vi "Main_Control_working.vi"() -> ()   [LabVIEW 2016]
panel:
  out "Workspace":T1(tab)
  in  "s_Path":path caption="Path"
  out "Scan":picture
  out "s_InkScape_path":string caption="String"
  in  "b_Change_litho":bool caption="Change"
  in  "l_Litho_modes":i32(ring) caption="Tip Signal Mode" items=["Current Measurement ", "Voltage Source", "Direct from BNC"]
  in  "b_Lithography_Mode":bool caption="Blank"
  in  "b_Open_InkScape":bool caption="Open"
  in  "b_Save_Scan":bool caption="Save"
  in  "b_Config":bool caption="Config"
  # "InkScape should open momentarily.\nHowever, if it fails to load in a reasonable amount of time, below is the path of the InkScape file if needed"
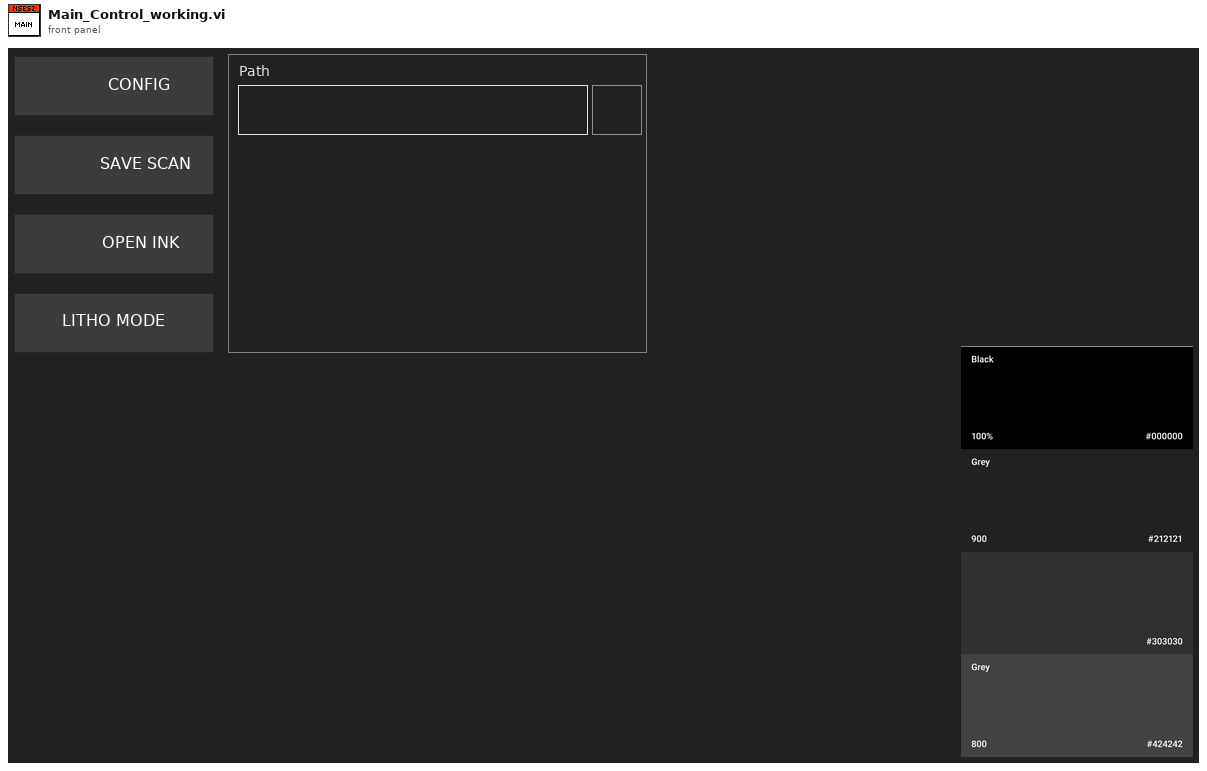
[diagram p1: front panel]
types:
  T1 = enum32{"CONFIG", "SAVE SCAN", "OPEN INKSCAPE", "LITHOMODE"}
  T2 = enum32{"invalid app kind", "Development System", "Run Time System", "Student Edition", "Embedded LabVIEW", "Evaluation", "Custom"}
  T3 = enum32{"Invalid", "Standard", "Closed", "Hidden", "Minimized", "Maximized"}
  T4 = cluster{"Core":cluster{"Current VI Reference":refnum<vi>, "Close Panel on Exit?":bool}, "Your Boolean data":bool, "Your string data":string, "Main_Path":path, "Image_Paths":cluster{"BMP":string, "BMP_Inkscape":string, "SVG_Inkscape":string}, "Application":refnum<k7>}
  T5 = cluster{"BMP":string, "BMP_Inkscape":string, "SVG_Inkscape":string}
  T6 = cluster{"Current VI Reference":refnum<vi>, "Close Panel on Exit?":bool}
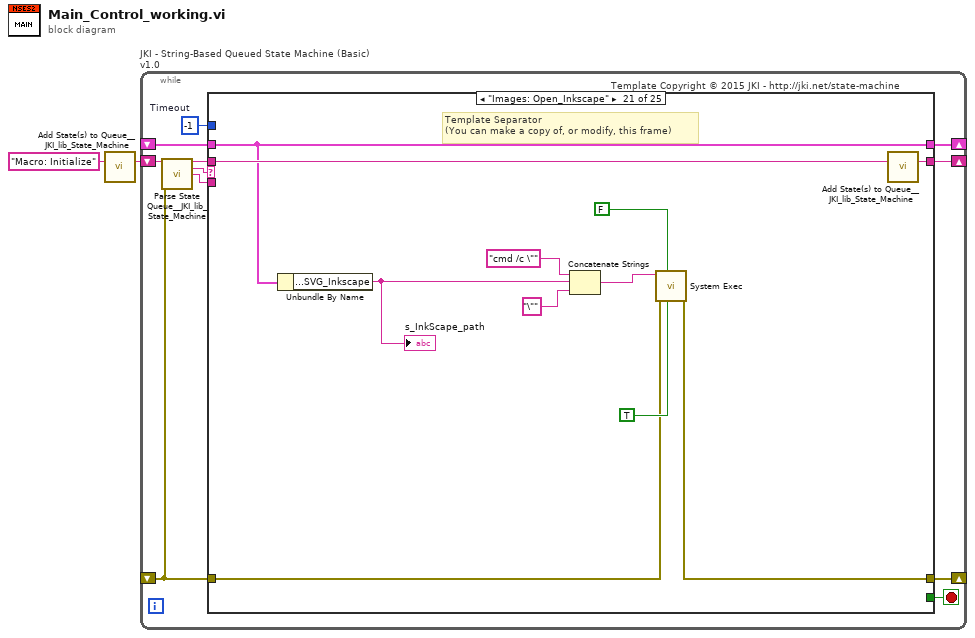
[diagram p0: block diagram]
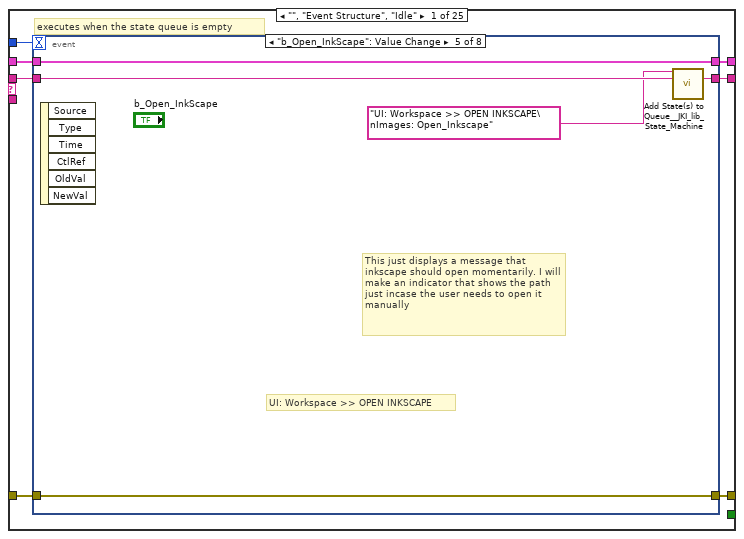
[diagram p2: hidden frame]
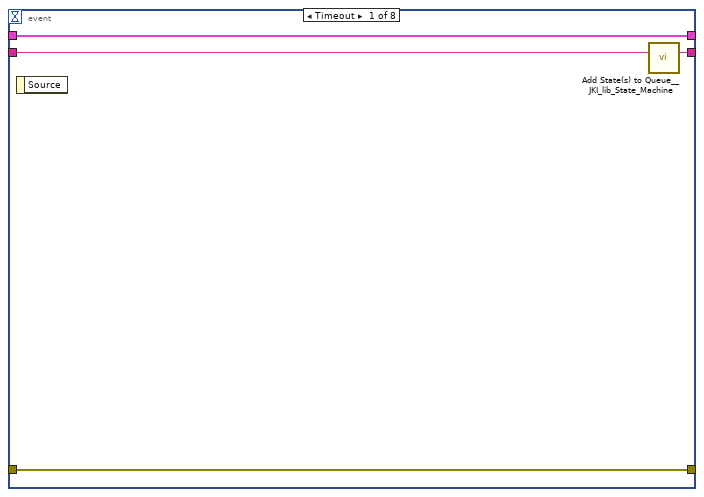
[diagram p3: hidden frame]
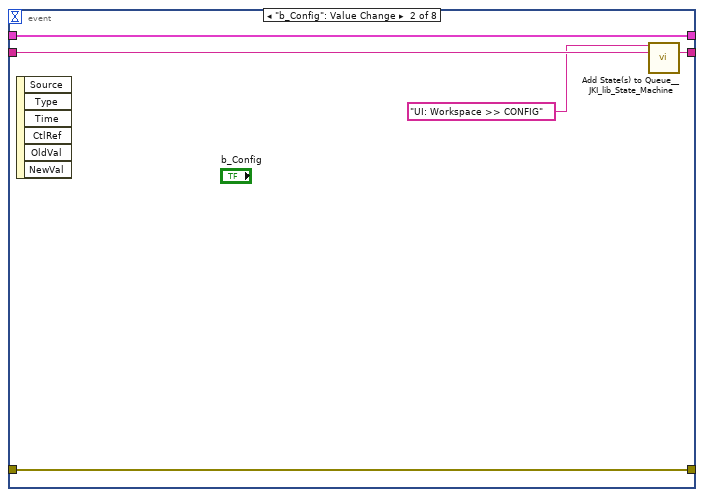
[diagram p4: hidden frame]
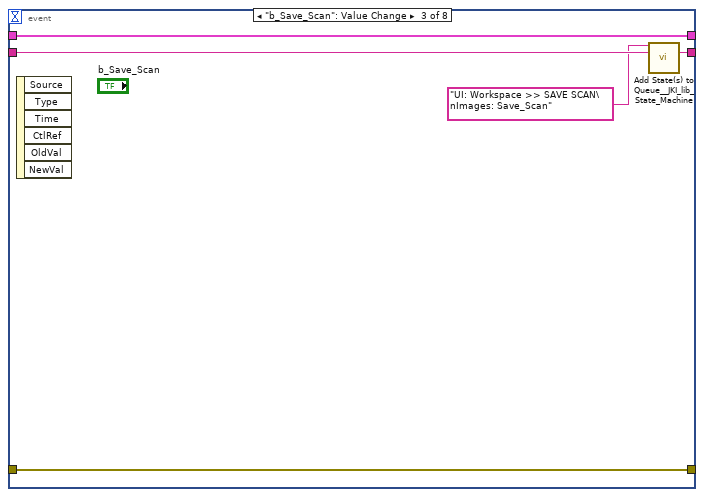
[diagram p5: hidden frame]
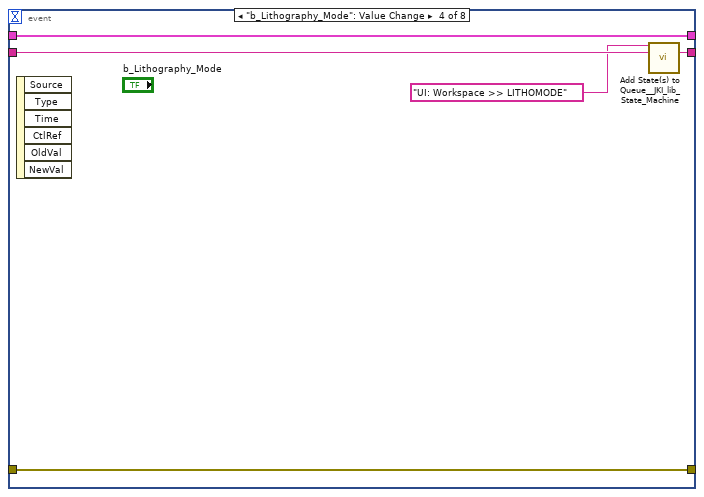
[diagram p6: hidden frame]
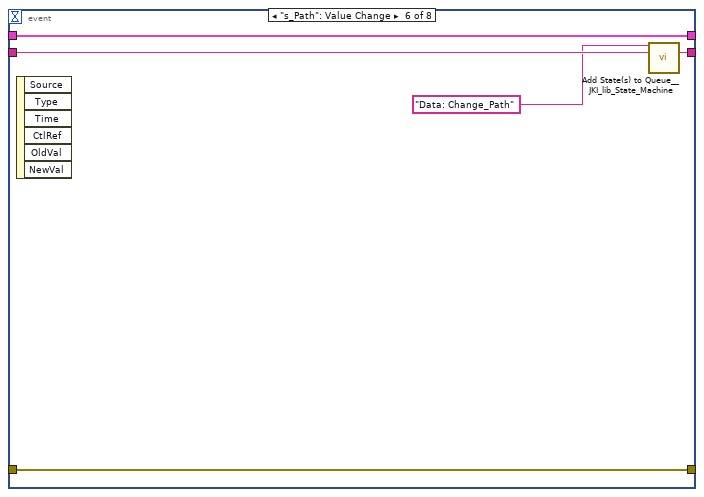
[diagram p7: hidden frame]
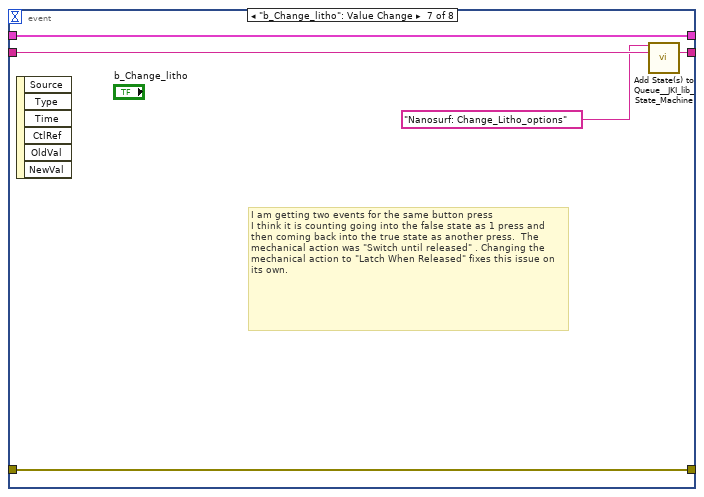
[diagram p8: hidden frame]
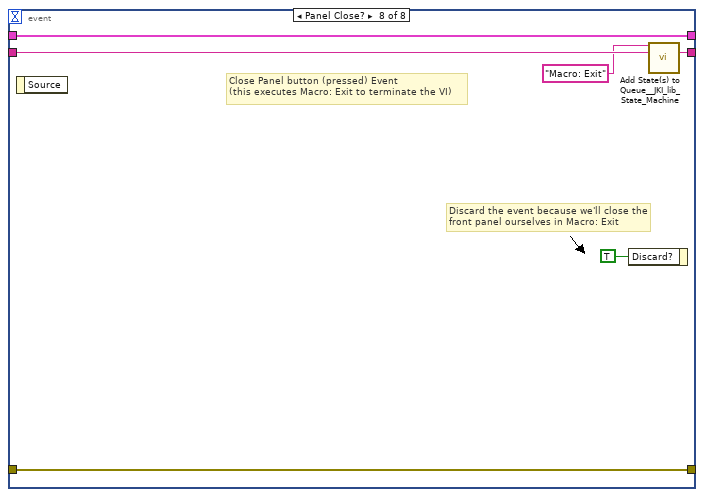
[diagram p9: hidden frame]
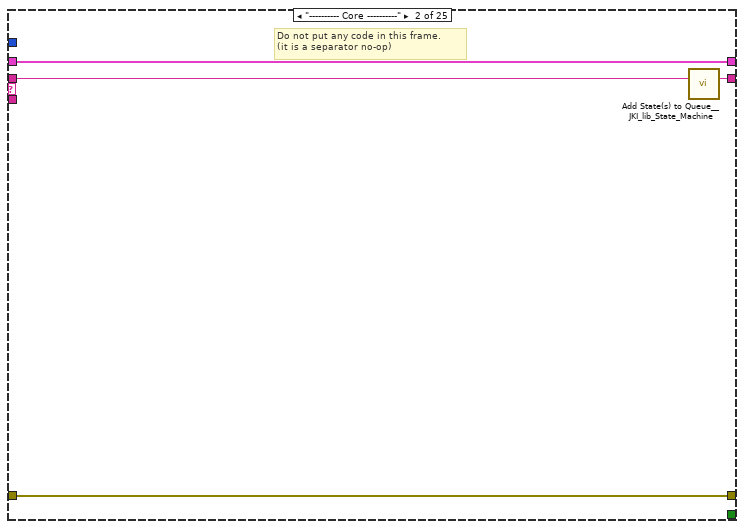
[diagram p10: hidden frame]
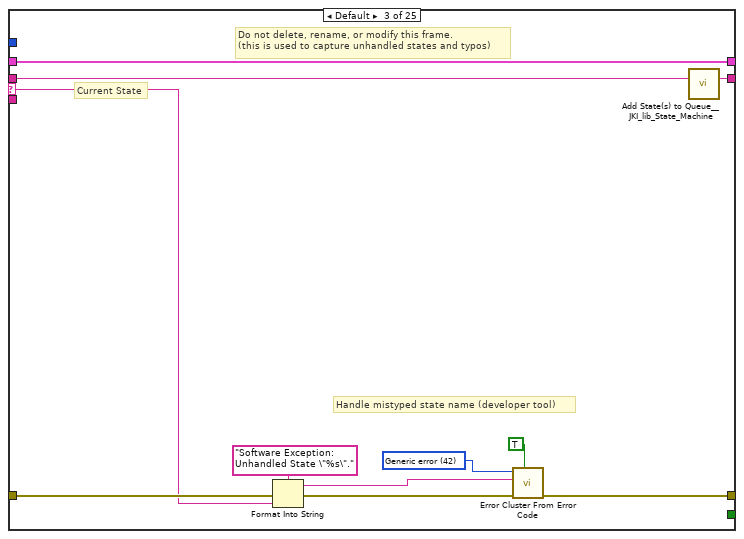
[diagram p11: hidden frame]
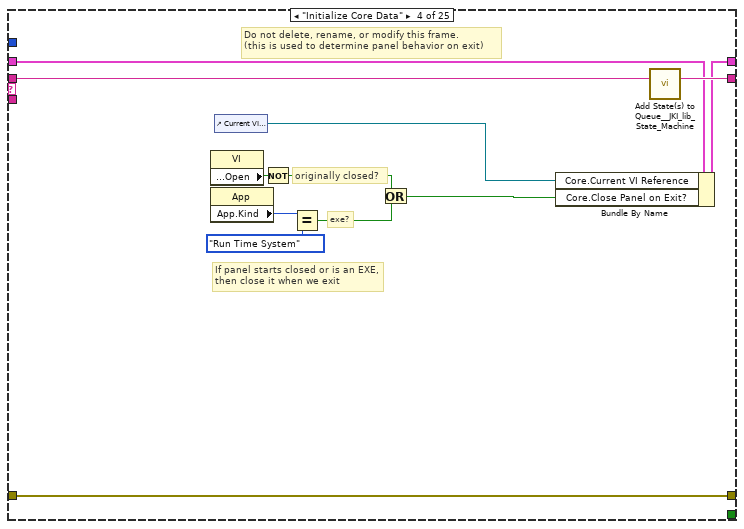
[diagram p12: hidden frame]
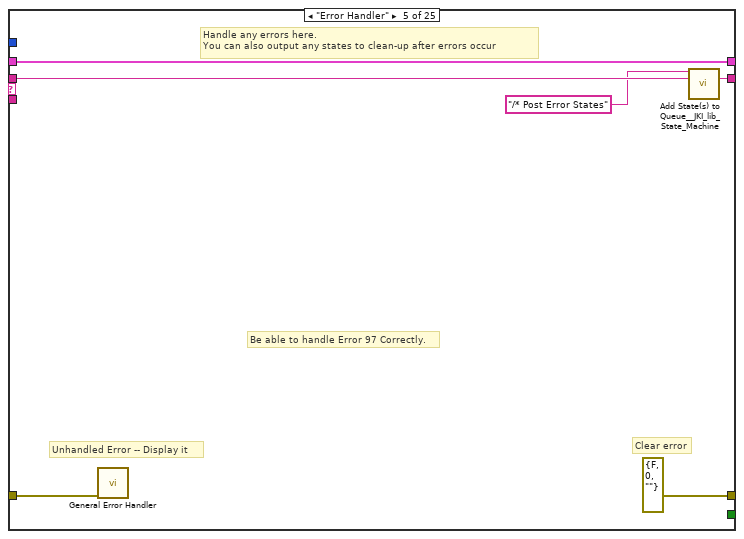
[diagram p13: hidden frame]
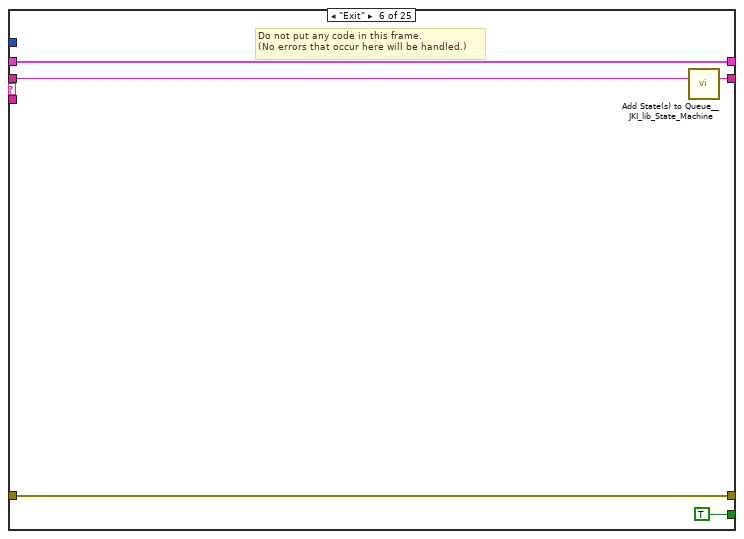
[diagram p14: hidden frame]
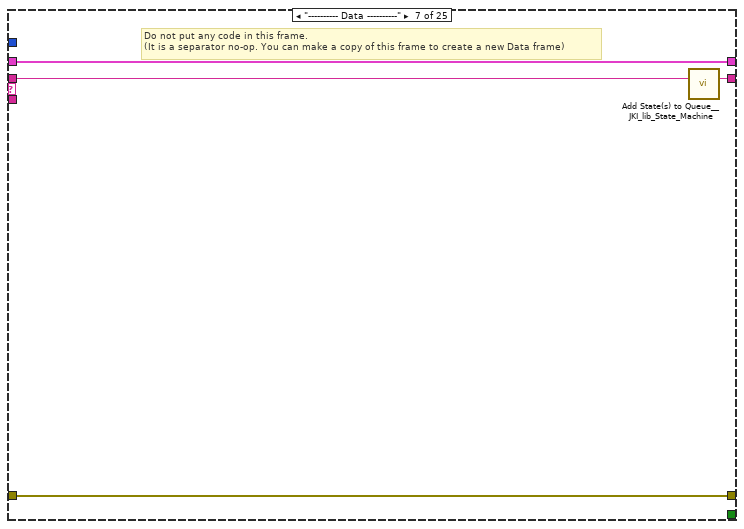
[diagram p15: hidden frame]
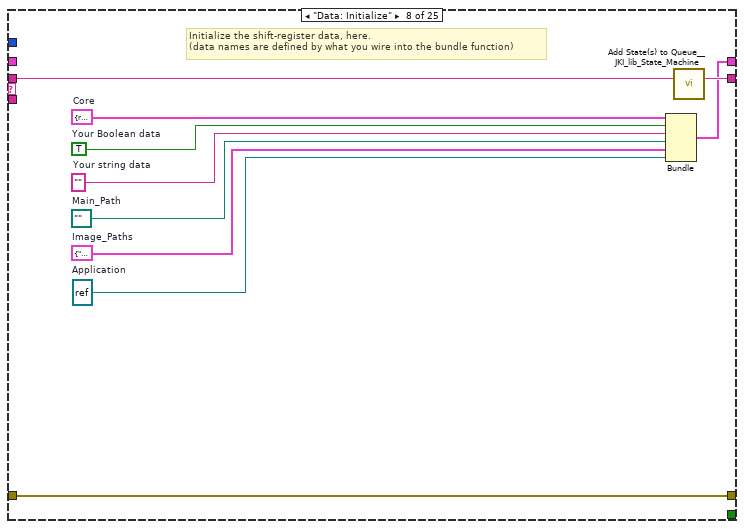
[diagram p16: hidden frame]
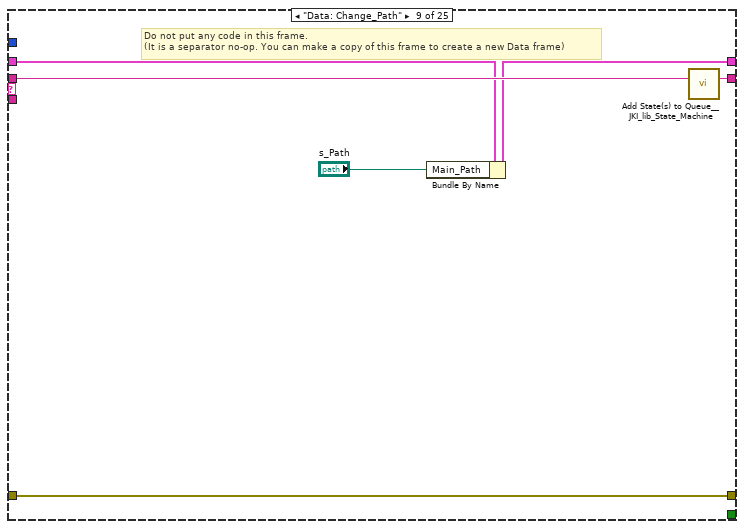
[diagram p17: hidden frame]
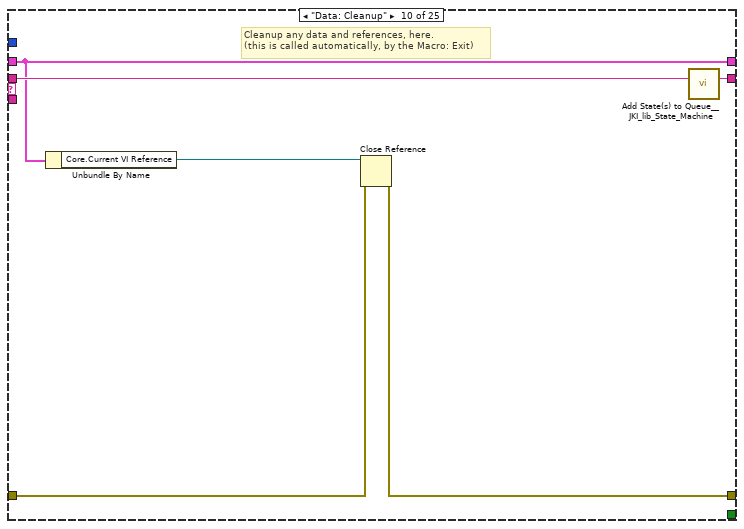
[diagram p18: hidden frame]
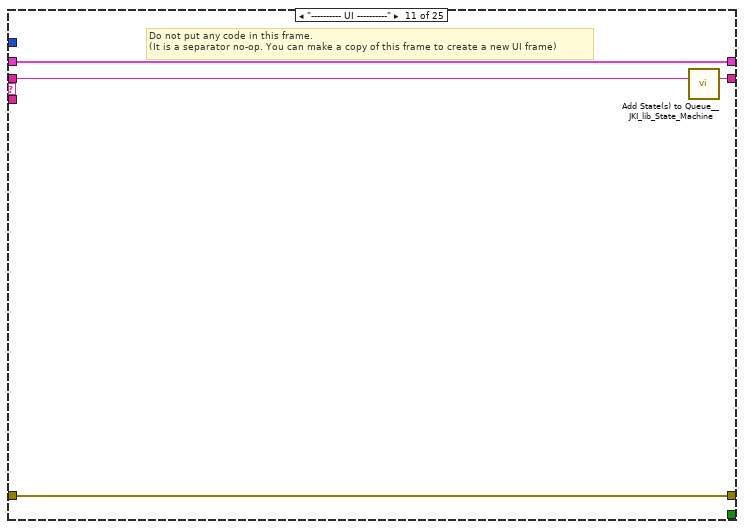
[diagram p19: hidden frame]
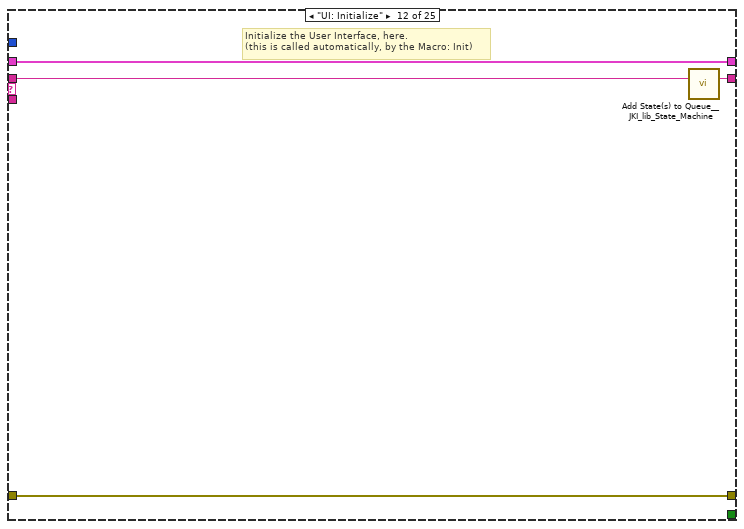
[diagram p20: hidden frame]
diagram:
  n1 = call <vilib>:"Add State(s) to Queue__JKI_lib_State_Machine.vi"("State(s) in (\"\")"="Macro: Initialize") -> ("States Out"=w2:string)  [unwired: 14 in]
  n2 = while "JKI - String-Based Queued State Machine (Basic) v1.0" {
    shift-right: [w6] -> _
    shift-left: _ -> [w5]
    shift-right: [w9] -> _
    shift-left: _ -> [w3]
    shift-right: [w8] -> _
    shift-left: w2 -> [w10]
    stop <- w7 stop-if-true
    w4 = -1  # Timeout
    # "Template Copyright © 2015 JKI - http://jki.net/state-machine"
    n3 = call <vilib>:"Parse State Queue__JKI_lib_State_Machine.vi"("State Queue"=w10, "Error In (no error)"=w3) -> ("Remaining States"=w12:string, "Current State"=w13:string, "Arguments"=w11:string)  [unwired: 11 in]
    n4 = case shown="\"Images: Open_Inkscape\"" w13 {
      selector: w13 -> [_ _ w65 _ _ _ _ _ _ _ _ _ _ _ _ _ _ _ _ _ _ _ _ _ _]
      tunnel: w12 -> [w20 w64 w69 w87 w93 w98 w102 w112 w118 w124 w128 w132 w138 w149 w177 w185 w190 w200 w204 w217 w228 w232 w240 w247 w253]
      tunnel: w11 -> [_ _ _ _ _ _ _ _ _ _ _ _ w133 w143 w173 _ _ _ _ _ _ _ _ _ _]
      tunnel: w5 -> [w18 w61 w67 w78 w90 w96 w99 _ w115 w119 w125 w130 w136 w145 w174 w182 w187 w197 w202 w210 w219 w229 w234 w245 w249]
      tunnel: [w17 w62 w71 w84 errorcluster {"status"=FALSE, "code"=0, "source"=""} ("error out") w95 w100 w109 w116 w120 w126 w129 w134 w146 w175 w183 w188 w198 w201 w213 w220 w230 w236 w241 w250] -> w9
      tunnel: w3 -> [w16 w62 w70 w84 w89 w95 w100 w109 w116 w121 w126 w129 w135 w147 w175 w183 w188 w198 w201 w214 w221 w230 w237 w242 w251]
      tunnel: [w19 w63 w68 w86 w92 w97 w101 w111 w117 w123 w127 w131 w137 w148 w176 w184 w189 w199 w203 w216 w227 w231 w239 w246 w252] -> w8
      tunnel: [_ _ _ _ _ TRUE _ _ _ _ _ _ _ _ _ _ _ _ _ _ _ _ _ _ _] -> w7
      tunnel: [w15 w61 w67 w85 w90 w96 w99 w110 w114 w119 w125 w130 w136 w145 w174 w182 w187 w197 w202 w209 w219 w229 w233 w245 w249] -> w6
      tunnel: w4 -> [w14 _ _ _ _ _ _ _ _ _ _ _ _ _ _ _ _ _ _ _ _ _ _ _ _]
      frame "", "Event Structure", "Idle" {
        # "executes when the state queue is empty"
        n5 = event shown="[4] \"b_Open_InkScape\": Value Change" {
          selector: _ -> [_ _ _ _ _ _ _ _]
          dyn-events: _ -> [_ _ _ _ _ _ _ _]
          timeout: w14 -> [_ _ _ _ _ _ _ _]
          tunnel: w20 -> [w24 w29 w34 w39 w44 w49 w54 w60]
          tunnel: [w23 w28 w33 w38 w43 w48 w53 w59] -> w19
          tunnel: w18 -> [w21 w26 w31 w36 w41 w46 w51 w57]
          tunnel: [w22 w27 w32 w37 w42 w47 w52 w58] -> w17
          tunnel: w16 -> [w22 w27 w32 w37 w42 w47 w52 w58]
          tunnel: [w21 w26 w31 w36 w41 w46 w51 w57] -> w15
          event Timeout {
            n6 = event-data() -> ()  [unwired: 1 in, 1 out]
            n7 = call <vilib>:"Add State(s) to Queue__JKI_lib_State_Machine.vi"("State(s) in (\"\")"=w24) -> ("States Out"=w23:string)  [unwired: 14 in]
          }
          event "b_Config": Value Change {
            n8 = event-data() -> ()  [unwired: 1 in, 6 out]
            n9 = call <vilib>:"Add State(s) to Queue__JKI_lib_State_Machine.vi"("State(s) in Front (\"\")"="UI: Workspace >> CONFIG" ("State(s) in Front (\"\")"), "State(s) in (\"\")"=w29) -> ("States Out"=w28:string)  [unwired: 13 in]
          }
          event "b_Save_Scan": Value Change {
            n10 = event-data() -> ()  [unwired: 1 in, 6 out]
            n11 = call <vilib>:"Add State(s) to Queue__JKI_lib_State_Machine.vi"("State(s) in Front (\"\")"="UI: Workspace >> SAVE SCAN\nImages: Save_Scan" ("State(s) in Front (\"\")"), "State(s) in (\"\")"=w34) -> ("States Out"=w33:string)  [unwired: 13 in]
          }
          event "b_Lithography_Mode": Value Change {
            n12 = event-data() -> ()  [unwired: 1 in, 6 out]
            n13 = call <vilib>:"Add State(s) to Queue__JKI_lib_State_Machine.vi"("State(s) in Front (\"\")"="UI: Workspace >> LITHOMODE" ("State(s) in Front (\"\")"), "State(s) in (\"\")"=w39) -> ("States Out"=w38:string)  [unwired: 13 in]
          }
          event "b_Open_InkScape": Value Change {
            # "This just displays a message that inkscape should open momentarily. I will make an indicator that shows the path just incase the user needs to open it manually"
            # "UI: Workspace >> OPEN INKSCAPE"
            n14 = event-data() -> ()  [unwired: 1 in, 6 out]
            n15 = call <vilib>:"Add State(s) to Queue__JKI_lib_State_Machine.vi"("State(s) in Front (\"\")"="UI: Workspace >> OPEN INKSCAPE\nImages: Open_Inkscape" ("State(s) in Front (\"\")"), "State(s) in (\"\")"=w44) -> ("States Out"=w43:string)  [unwired: 13 in]
          }
          event "s_Path": Value Change {
            n16 = event-data() -> ()  [unwired: 1 in, 6 out]
            n17 = call <vilib>:"Add State(s) to Queue__JKI_lib_State_Machine.vi"("State(s) in Front (\"\")"="Data: Change_Path" ("State(s) in Front (\"\")"), "State(s) in (\"\")"=w49) -> ("States Out"=w48:string)  [unwired: 13 in]
          }
          event "b_Change_litho": Value Change {
            # "I am getting two events for the same button press \nI think it is counting going into the false state as 1 press and then coming back into the true state as another press.  The mechanical action was \"Switch until released\" . Changing the mechanical action to \"Latch When Released\" fixes this issue on its own."
            n18 = event-data() -> ()  [unwired: 1 in, 6 out]
            n19 = call <vilib>:"Add State(s) to Queue__JKI_lib_State_Machine.vi"("State(s) in Front (\"\")"="Nanosurf: Change_Litho_options", "State(s) in (\"\")"=w54) -> ("States Out"=w53:string)  [unwired: 13 in]
          }
          event Panel Close? {
            # "Discard the event because we'll close the front panel ourselves in Macro: Exit"
            # "Close Panel button (pressed) Event\n(this executes Macro: Exit to terminate the VI)"
            n20 = event-data() -> ()  [unwired: 1 in, 1 out]
            n21 = event-data("Discard?"=TRUE) -> ()  [unwired: 1 in, 1 out]
            n22 = call <vilib>:"Add State(s) to Queue__JKI_lib_State_Machine.vi"("State(s) in Front (\"\")"="Macro: Exit", "State(s) in (\"\")"=w60) -> ("States Out"=w59:string)  [unwired: 13 in]
          }
        }
      }
      frame "---------- Core ----------" {
        # "Do not put any code in this frame.\n(it is a separator no-op)"
        n23 = call <vilib>:"Add State(s) to Queue__JKI_lib_State_Machine.vi"("State(s) in (\"\")"=w64) -> ("States Out"=w63:string)  [unwired: 14 in]
      }
      frame Default {
        w74 = 42 items=["No error", "Argument error", "Memory is full", "Out of zone", "End of file", "File already open", "Generic file I/O error", "File not found", "File permission error", "Disk is full", "Duplicate path", "Too many files open", "System feature not enabled", "Resource file not found", "Cannot add resource", "Resource not found", "Image not found", "Image memory error", "Pen does not exist", "Config type invalid", "Config token not found", "Config parse error", "Config memory error", "Bad external code format", "Bad external code offset", "External code not present", "Null window", "Destroy window error", "Null menu", "Print aborted", "Bad print record", "Print driver error", "Windows error during printing", "Memory error during printing", "Print dialog error", "Generic print error", "Invalid device refnum", "Device not found", "Device parameter error", "Device unit error", "Cannot open device", "Device call aborted", "Generic error", "Cancelled by user", "Object ID too low", "Object ID too high", "Object not in heap", "Unknown heap", "Unknown object (invalid DefProc)", "Unknown object (DefProc not in table)", "Message out of range", "Invalid (null) method", "Unknown message", "Manager call not supported", "Bad address", "Network operation in progress", "Network operation timed out", "Connection is busy", "Network attribute not supported", "Network error", "Address in use", "System out of memory", "Connection aborted", "Connection refused", "Not connected", "Already connected", "Connection closed", "Initialization error (interapplication manager)", "Bad occurrence", "Wait on unbound occurrence handler", "Occurrence queue overflow", "Datalog type conflict", "Unused", "Unrecognized type (interapplication manager)", "Memory corrupt", "Failed to make temporary DLL", "Old CIN version", "Drag socket not found", "Failed to load drop-object", "Failed to register OLE object", "Failed to release OLE object", "Format specifier type mismatch", "Unknown format specifier", "Too few format specifiers", "Too many format specifiers", "Scan failed", "Newer CIN version", "Error converting to variant", "Runtime menu error", "Password tampered", "Variant attribute not found", "Incompatible variant data type", "Event data is not available", "Event Store is not present", "Occurrence is not found", "Event Queue is not created", "Event info is not available", "Refnum passed is NULL", "Error retrieving Class GUID", "Error retrieving CoClass GUID", "Error retrieving TypeLib GUID.", "Bad built application magic bytes.", "Specific driver is different from the specific driver associated with the Logical Name.", "There is no session opened to the class driver.", "Max Error", "MAX - Error with config objects", "MAX - Error loading configuration", "MAX - Group not supported"]
        # "Current State"
        # "Do not delete, rename, or modify this frame.\n(this is used to capture unhandled states and typos)"
        # "Handle mistyped state name (developer tool)"
        n24 = Format Into String(format string="Software Exception: Unhandled State \"%s\"." ("message"), error in=w70, w65) -> (resulting string=w73:string, error out=w72:errorcluster)  [unwired: 1 in]
        n25 = call <vilib>:"Error Cluster From Error Code.vi"("show call chain? (False)"=TRUE, "error in (no error)"=w72, "error message (\"\")"=w73, "error code (0)"=w74) -> ("error out"=w71:errorcluster)  [unwired: 5 in]
        n26 = call <vilib>:"Add State(s) to Queue__JKI_lib_State_Machine.vi"("State(s) in (\"\")"=w69) -> ("States Out"=w68:string)  [unwired: 14 in]
      }
      frame "Initialize Core Data" {
        # "Do not delete, rename, or modify this frame.\n(this is used to determine panel behavior on exit)"
        # "originally closed?"
        # "exe?"
        # "If panel starts closed or is an EXE, then close it when we exit"
        n27 = property class="VI"() -> ("Front Panel.Open"=w83:bool)  [unwired: 2 in, 2 out]
        n28 = property class="App"() -> ("App.Kind"=w82:T2)  [unwired: 2 in, 2 out]
        n29 = control-ref of="Current VI Reference"() -> (w76:refnum<vi>)
        n30 = Not(x=w83) -> (.not. x?=w80:bool)
        n31 = Equal?(x=w82, y=T2."Run Time System" ("Application:Kind")) -> (x = y?=w79:bool)
        n32 = Or(x=w80, y=w79) -> (x .or. y?=w77:bool)
        n33 = Bundle By Name(cluster=w78, "Core.Current VI Reference"=w76, "Core.Close Panel on Exit?"=w77) -> (w85:T4)
        n34 = call <vilib>:"Add State(s) to Queue__JKI_lib_State_Machine.vi"("State(s) in (\"\")"=w87) -> ("States Out"=w86:string)  [unwired: 14 in]
      }
      frame "Error Handler" {
        # "Be able to handle Error 97 Correctly."
        # "Unhandled Error -- Display it"
        # "Handle any errors here.\nYou can also output any states to clean-up after errors occur"
        # "Clear error"
        n35 = call <vilib>:"General Error Handler.vi"("error in (no error)"=w89) -> ()  [unwired: 10 in, 5 out]
        n36 = call <vilib>:"Add State(s) to Queue__JKI_lib_State_Machine.vi"("State(s) in Front (\"\")"="/* Post Error States", "State(s) in (\"\")"=w93) -> ("States Out"=w92:string)  [unwired: 13 in]
      }
      frame "Exit" {
        # "Do not put any code in this frame.\n(No errors that occur here will be handled.)"
        n37 = call <vilib>:"Add State(s) to Queue__JKI_lib_State_Machine.vi"("State(s) in (\"\")"=w98) -> ("States Out"=w97:string)  [unwired: 14 in]
      }
      frame "---------- Data ----------" {
        # "Do not put any code in this frame.\n(It is a separator no-op. You can make a copy of this frame to create a new Data frame)"
        n38 = call <vilib>:"Add State(s) to Queue__JKI_lib_State_Machine.vi"("State(s) in (\"\")"=w102) -> ("States Out"=w101:string)  [unwired: 14 in]
      }
      frame "Data: Initialize" {
        w103 = refnum<k7> refnum  # Application
        w104 = T5 {"BMP"="", "BMP_Inkscape"="", "SVG_Inkscape"=""}  # Image_Paths
        w105 = path ""  # Main_Path
        w106 = T6 {"Current VI Reference"=refnum, "Close Panel on Exit?"=FALSE}  # Core
        w108 = TRUE  # Your Boolean data
        w107 = ""  # Your string data
        # "Initialize the shift-register data, here.\n(data names are defined by what you wire into the bundle function)"
        n39 = Bundle("Core"=w106, "Your Boolean data"=w108, "Your string data"=w107, "Main_Path"=w105, "Image_Paths"=w104, "Application"=w103) -> (w110:T4)  [unwired: 1 in]
        n40 = call <vilib>:"Add State(s) to Queue__JKI_lib_State_Machine.vi"("State(s) in (\"\")"=w112) -> ("States Out"=w111:string)  [unwired: 14 in]
      }
      frame "Data: Change_Path" {
        # "Do not put any code in this frame.\n(It is a separator no-op. You can make a copy of this frame to create a new Data frame)"
        n41 = Bundle By Name(cluster=w115, "Main_Path"="s_Path") -> (w114:T4)
        n42 = call <vilib>:"Add State(s) to Queue__JKI_lib_State_Machine.vi"("State(s) in (\"\")"=w118) -> ("States Out"=w117:string)  [unwired: 14 in]
      }
      frame "Data: Cleanup" {
        # "Cleanup any data and references, here.\n(this is called automatically, by the Macro: Exit)"
        n43 = Unbundle By Name(w119) -> ("Core.Current VI Reference"=w122:refnum<vi>)
        n44 = Close Reference(reference=w122, error in (no error)=w121) -> (error out=w120:errorcluster)
        n45 = call <vilib>:"Add State(s) to Queue__JKI_lib_State_Machine.vi"("State(s) in (\"\")"=w124) -> ("States Out"=w123:string)  [unwired: 14 in]
      }
      frame "---------- UI ----------" {
        # "Do not put any code in this frame.\n(It is a separator no-op. You can make a copy of this frame to create a new UI frame)"
        n46 = call <vilib>:"Add State(s) to Queue__JKI_lib_State_Machine.vi"("State(s) in (\"\")"=w128) -> ("States Out"=w127:string)  [unwired: 14 in]
      }
      frame "UI: Initialize" {
        # "Initialize the User Interface, here.\n(this is called automatically, by the Macro: Init)"
        n47 = call <vilib>:"Add State(s) to Queue__JKI_lib_State_Machine.vi"("State(s) in (\"\")"=w132) -> ("States Out"=w131:string)  [unwired: 14 in]
      }
      frame "UI: Cursor Set" {
        # "Argument"
        # "Set and Unset Cursor Busy.\n(Usage: \"UI: Cursor Set >> Busy|Idle\")"
        n48 = case shown="\"Idle\", Default" w133 {
          tunnel: w135 -> [w140 w142]
          tunnel: [w139 w141] -> w134
          frame "Idle", Default {
            n49 = call <vilib>:"Unset Busy.vi"("error in (no error)"=w140) -> ("error out"=w139:errorcluster)  [unwired: 10 in]
          }
          frame "Busy" {
            n50 = call <vilib>:"Set Busy.vi"("error in (no error)"=w142) -> ("error out"=w141:errorcluster)  [unwired: 9 in, 1 out]
          }
        }
        n51 = call <vilib>:"Add State(s) to Queue__JKI_lib_State_Machine.vi"("State(s) in (\"\")"=w138) -> ("States Out"=w137:string)  [unwired: 14 in]
      }
      frame "UI: Front Panel State" {
        # "Argument"
        # "Set Front Panel Open or Closed\n(Usage: \"UI: Front Panel State >> Open|Close\")"
        n52 = Unbundle By Name(w145) -> ("Core.Current VI Reference"=w144:refnum<vi>)
        n53 = case shown="\"Open\", Default" w143 {
          tunnel: w147 -> [w153 w166]
          tunnel: [w155 w167] -> w146
          tunnel: w144 -> [w154 w164]
          frame "Open", Default {
            n54 = property class="VI"(reference=w154, error in=w153) -> (reference out=w151:refnum<vi>, error out=w152:errorcluster, "Front Panel.Open"=w150:bool)
            n55 = case shown="False" w150 {
              tunnel: [w158 w161] -> w155
              tunnel: w152 -> [w157 w161]
              tunnel: w151 -> [w156 _]
              frame False {
                n56 = invoke class="VI" method="FP.Open"(reference=w156, error in=w157, "Activate"=TRUE, "State"=T3."Standard") -> (error out=w158:errorcluster)  [unwired: 1 in, 4 out]
              }
              frame True {
              }
            }
          }
          frame "Close" {
            n57 = property class="VI"(reference=w164, error in=w166) -> (reference out=w163:refnum<vi>, error out=w165:errorcluster, "Front Panel.Open"=w162:bool)
            n58 = case shown="True" w162 {
              tunnel: [w168 w171] -> w167
              tunnel: w165 -> [w168 w170]
              tunnel: w163 -> [_ w169]
              frame False {
              }
              frame True {
                n59 = invoke class="VI" method="FP.Close"(reference=w169, error in=w170) -> (error out=w171:errorcluster)  [unwired: 1 in, 2 out]
              }
            }
          }
        }
        n60 = call <vilib>:"Add State(s) to Queue__JKI_lib_State_Machine.vi"("State(s) in (\"\")"=w149) -> ("States Out"=w148:string)  [unwired: 14 in]
      }
      frame "UI: Workspace" {
        # "Workspace Tab State\n(This is the frame that changes the Workspace Value)"
        n61 = case shown="\"OPEN INKSCAPE\"" w173 {
          tunnel: [T1."CONFIG" ("Workspace") T1."SAVE SCAN" ("Workspace") T1."OPEN INKSCAPE" ("Workspace") T1."LITHOMODE" ("Workspace")] -> w172
          frame "CONFIG", Default {
            # "UI: Workspace >> CONFIG"
          }
          frame "SAVE SCAN" {
            # "UI: Workspace >> SAVE SCAN"
          }
          frame "OPEN INKSCAPE" {
            # "UI: Workspace >> OPEN INKSCAPE"
          }
          frame "LITHOMODE" {
            # "UI: Workspace >> LITHOMODE"
          }
        }
        "Workspace" <- w172
        n62 = call <vilib>:"Add State(s) to Queue__JKI_lib_State_Machine.vi"("State(s) in (\"\")"=w177) -> ("States Out"=w176:string)  [unwired: 14 in]
      }
      frame "---------- Macro ----------" {
        # "Do not put any code in this frame.\n(It is a separator no-op. You can make a copy of this frame to create a new Macro frame)"
        n63 = call <vilib>:"Add State(s) to Queue__JKI_lib_State_Machine.vi"("State(s) in (\"\")"=w185) -> ("States Out"=w184:string)  [unwired: 14 in]
      }
      frame "Macro: Initialize" {
        w186 = "Data: Initialize\nInitialize Core Data\nUI: Initialize\nUI: Front Panel State >> Open\nUI: Workspace >> CONFIG\nNanosurf: Open_Application\nData: Change_Path"  # Data: Initialize Initialize Core Data UI: Initialize UI: Front Panel State >> Open UI: Workspace >> CONFIG Nanosurf: Open_Application Data: Change_Path
        # "Initialization Macro\n(This is called once, when the VI starts)"
        n64 = call <vilib>:"Add State(s) to Queue__JKI_lib_State_Machine.vi"("State(s) in Front (\"\")"=w186, "State(s) in (\"\")"=w190) -> ("States Out"=w189:string)  [unwired: 13 in]
      }
      frame "Macro: Exit" {
        # "Exit Macro\n(This is called once, when the VI exits)"
        n65 = Unbundle By Name(w197) -> ("Core.Close Panel on Exit?"=w196:bool)
        n66 = Select(t="UI: Front Panel State >> Close", s=w196, f="") -> (s? t:f=w193:string)
        n67 = call <vilib>:"Add State(s) to Queue__JKI_lib_State_Machine.vi"("State(s) in (\"\")"=w193, "State(s) at Back (\"\")"="UI: Workspace >> CONFIG\nNanosurf: Close_Application\nData: Cleanup\nExit") -> ("States Out"=w191:string)  [unwired: 13 in]
        n68 = call <vilib>:"Add State(s) to Queue__JKI_lib_State_Machine.vi"("State(s) in Front (\"\")"=w191, "State(s) in (\"\")"=w200) -> ("States Out"=w199:string)  [unwired: 13 in]
      }
      frame "---------- Images ----------" {
        # "Template Separator\n(You can make a copy of, or modify, this frame)"
        n69 = call <vilib>:"Add State(s) to Queue__JKI_lib_State_Machine.vi"("State(s) in (\"\")"=w204) -> ("States Out"=w203:string)  [unwired: 14 in]
      }
      frame "Images: Save_Scan" {
        # "Template Separator\n(This will make an make a copy of, or modify, this frame)"
        n70 = Unbundle By Name(w210) -> ("Application"=w205:refnum<k7>, "Main_Path"=w211:path)
        n71 = call "Generic file paths.vi"("error in (no error)"=w214, "Parent Folder"=w211) -> ("error out"=w215:errorcluster, "SVG Path"=w206:string, "BMP for inkscape path"=w207:string, "BMP Path"=w208:string)  [unwired: 6 in]
        n72 = call "Save_Scan_macro.vi"("Application"=w205, "error in (no error)"=w215, "InkScape"=w206, "BMP INK Path"=w207, "BMP Path"=w208) -> ("error out"=w213:errorcluster, "BMP"=→"Scan":picture)  [unwired: 5 in]
        n73 = Bundle By Name(cluster=w210, "Image_Paths.BMP"=w208, "Image_Paths.BMP_Inkscape"=w207, "Image_Paths.SVG_Inkscape"=w206) -> (w209:T4)
        n74 = call <vilib>:"Add State(s) to Queue__JKI_lib_State_Machine.vi"("State(s) in (\"\")"=w217) -> ("States Out"=w216:string)  [unwired: 14 in]
      }
      frame "Images: Open_Inkscape" {
        # "Template Separator\n(You can make a copy of, or modify, this frame)"
        n75 = Unbundle By Name(w219) -> ("Image_Paths.SVG_Inkscape"=w218:string)
        "s_InkScape_path" <- w218
        n76 = Concatenate Strings("cmd /c \"", w218, "\"") -> (w224:string)
        n77 = call <vilib>:"System Exec.vi"("run minimized? (F)"=TRUE, "wait until completion? (T)"=FALSE, "error in (no error)"=w221, "command line"=w224) -> ("error out"=w220:errorcluster)  [unwired: 4 in, 3 out]
        n78 = call <vilib>:"Add State(s) to Queue__JKI_lib_State_Machine.vi"("State(s) in (\"\")"=w228) -> ("States Out"=w227:string)  [unwired: 14 in]
      }
      frame "---------- Nanosurf ----------" {
        # "Template Separator\n(You can make a copy of, or modify, this frame)"
        n79 = call <vilib>:"Add State(s) to Queue__JKI_lib_State_Machine.vi"("State(s) in (\"\")"=w232) -> ("States Out"=w231:string)  [unwired: 14 in]
      }
      frame "Nanosurf: Open_Application" {
        n80 = Unbundle By Name(w234) -> ("Application"=w238:refnum<k7>)
        n81 = Automation Open(error in (no error)=w237, Automation Refnum=w238) -> (Automation Refnum=w235:refnum<k7>, error out=w236:errorcluster)  [unwired: 2 in]
        n82 = Bundle By Name(cluster=w234, "Application"=w235) -> (w233:T4)
        n83 = call <vilib>:"Add State(s) to Queue__JKI_lib_State_Machine.vi"("State(s) in (\"\")"=w240) -> ("States Out"=w239:string)  [unwired: 14 in]
      }
      frame "Nanosurf: Change_Litho_options" {
        # "Change Lithography Options\n(Changes what the microscope uses to source the tip voltage. [more options may be added later])"
        n84 = Unbundle By Name(w245) -> ("Application"=w244:refnum<k7>)
        n85 = call "Change_tip_signal.vi"("error in (no error)"=w242, "l_Litho_modes"="l_Litho_modes", "Application"=w244) -> ("error out"=w241:errorcluster)  [unwired: 8 in]
        n86 = call <vilib>:"Add State(s) to Queue__JKI_lib_State_Machine.vi"("State(s) in (\"\")"=w247) -> ("States Out"=w246:string)  [unwired: 14 in]
      }
      frame "Nanosurf: Close_Application" {
        # "Template Separator\n(You can make a copy of, or modify, this frame)"
        n87 = Unbundle By Name(w249) -> ("Application"=w248:refnum<k7>)
        n88 = Close Reference(reference=w248, error in (no error)=w251) -> (error out=w250:errorcluster)
        n89 = call <vilib>:"Add State(s) to Queue__JKI_lib_State_Machine.vi"("State(s) in (\"\")"=w253) -> ("States Out"=w252:string)  [unwired: 14 in]
      }
    }
  }
